vi "SaveBlock.vi"(6 "Registry":T13, 7 "start block":T21, 8 "error in (no error)":errorcluster, 9 "data":T9, 10 "data event config":T17, 11 "data event":T1) -> (0 "error out":errorcluster, 1 "file complete":bool, 2 "data event config out":T17, 3 "data event out":T1)   [LabVIEW 2017, in "CmsDataEventCreator.lvlib"]
uses:
  <vilib>/addons/InsightCM/Devices/Shared/Cms/CmsDataEventCreator/CmsDataEventCreator.lvlib
  <vilib>/addons/InsightCM/Devices/Shared/Common/DVRBuffer/controls/BufferLocation.ctl
  <vilib>/addons/InsightCM/Devices/Shared/Cms/CmsDataEventCreator/controls/DataEventConfig.ctl
  <vilib>/addons/InsightCM/Devices/Shared/Cms/CmsDataEventCreator/controls/AcqParams.ctl
  <vilib>/addons/InsightCM/Devices/Shared/Common/DataAccumulator/controls/AccumulationSettings.ctl
  <vilib>/addons/InsightCM/Devices/Shared/Common/DataAccumulator/controls/accumulationType.ctl
  <vilib>/addons/PointValueMap/controls/PointMap.ctl
  <vilib>/addons/InsightCM/Devices/Shared/Cms/CmsDataEventCreator/controls/GroupRegistry.ctl
  <vilib>/addons/InsightCM/Devices/Shared/Cms/CmsDataEventCreator/controls/DataSetRegistry.ctl
  <vilib>/addons/InsightCM/Devices/Shared/Common/DataEvent/controls/DataSetType.ctl
  <vilib>/addons/InsightCM/Devices/Shared/Common/DataEventCreator/controls/Registry_Trend.ctl
  <vilib>/addons/InsightCM/Devices/Shared/Common/DataFlow/controls/Data.ctl
  <vilib>/addons/InsightCM/Utilities/DataAccessors/controls/wfmSGL_DVR.ctl
  <vilib>/addons/InsightCM/Devices/Shared/Common/DataFlow/controls/Type.ctl
  <vilib>/addons/InsightCM/Devices/Shared/Common/DataEvent/controls/Event.ctl
  <vilib>/addons/InsightCM/MessageBus/Base/controls/DataEvent.ctl
  <vilib>/addons/InsightCM/MessageBus/Base/controls/KeyValuePair.ctl
  <vilib>/addons/InsightCM/Devices/Shared/Common/DataEvent/controls/DataSet.ctl
  <vilib>/addons/InsightCM/MessageBus/Base/controls/DataSetMetadata.ctl
  <vilib>/addons/InsightCM/MessageBus/Base/controls/TrendPoint.ctl
  <vilib>/addons/InsightCM/MessageBus/Base/controls/TrendAlarmUpdate.ctl
  <vilib>/addons/InsightCM/MessageBus/Base/controls/TrendAlarmTransition.ctl
  <vilib>/addons/InsightCM/Devices/Shared/Common/DataAccumulator/controls/DataStoreType.ctl
  <vilib>/addons/InsightCM/Utilities/Analysis/Shared/controls/PulsePositions.ctl
  <vilib>/addons/InsightCM/Devices/Shared/Common/DataAccumulator/DataAccumulator.lvlib
  <vilib>/addons/InsightCM/Utilities/Analysis/Shared/AnalysisHelper.lvlib
  <vilib>/addons/InsightCM/Devices/Shared/Common/DVRBuffer/DVRBuffer.lvlib
  <vilib>/addons/InsightCM/Devices/Shared/Common/DataFlow/DataFlow.lvlib
  <vilib>/addons/PointValueMap/PointValueMap.lvlib
  <vilib>/addons/InsightCM/Devices/Shared/Common/DataEvent/DataEvent.lvlib
  <vilib>/addons/InsightCM/Devices/Shared/Common/DataEventCreator/DataEventCreator.lvlib
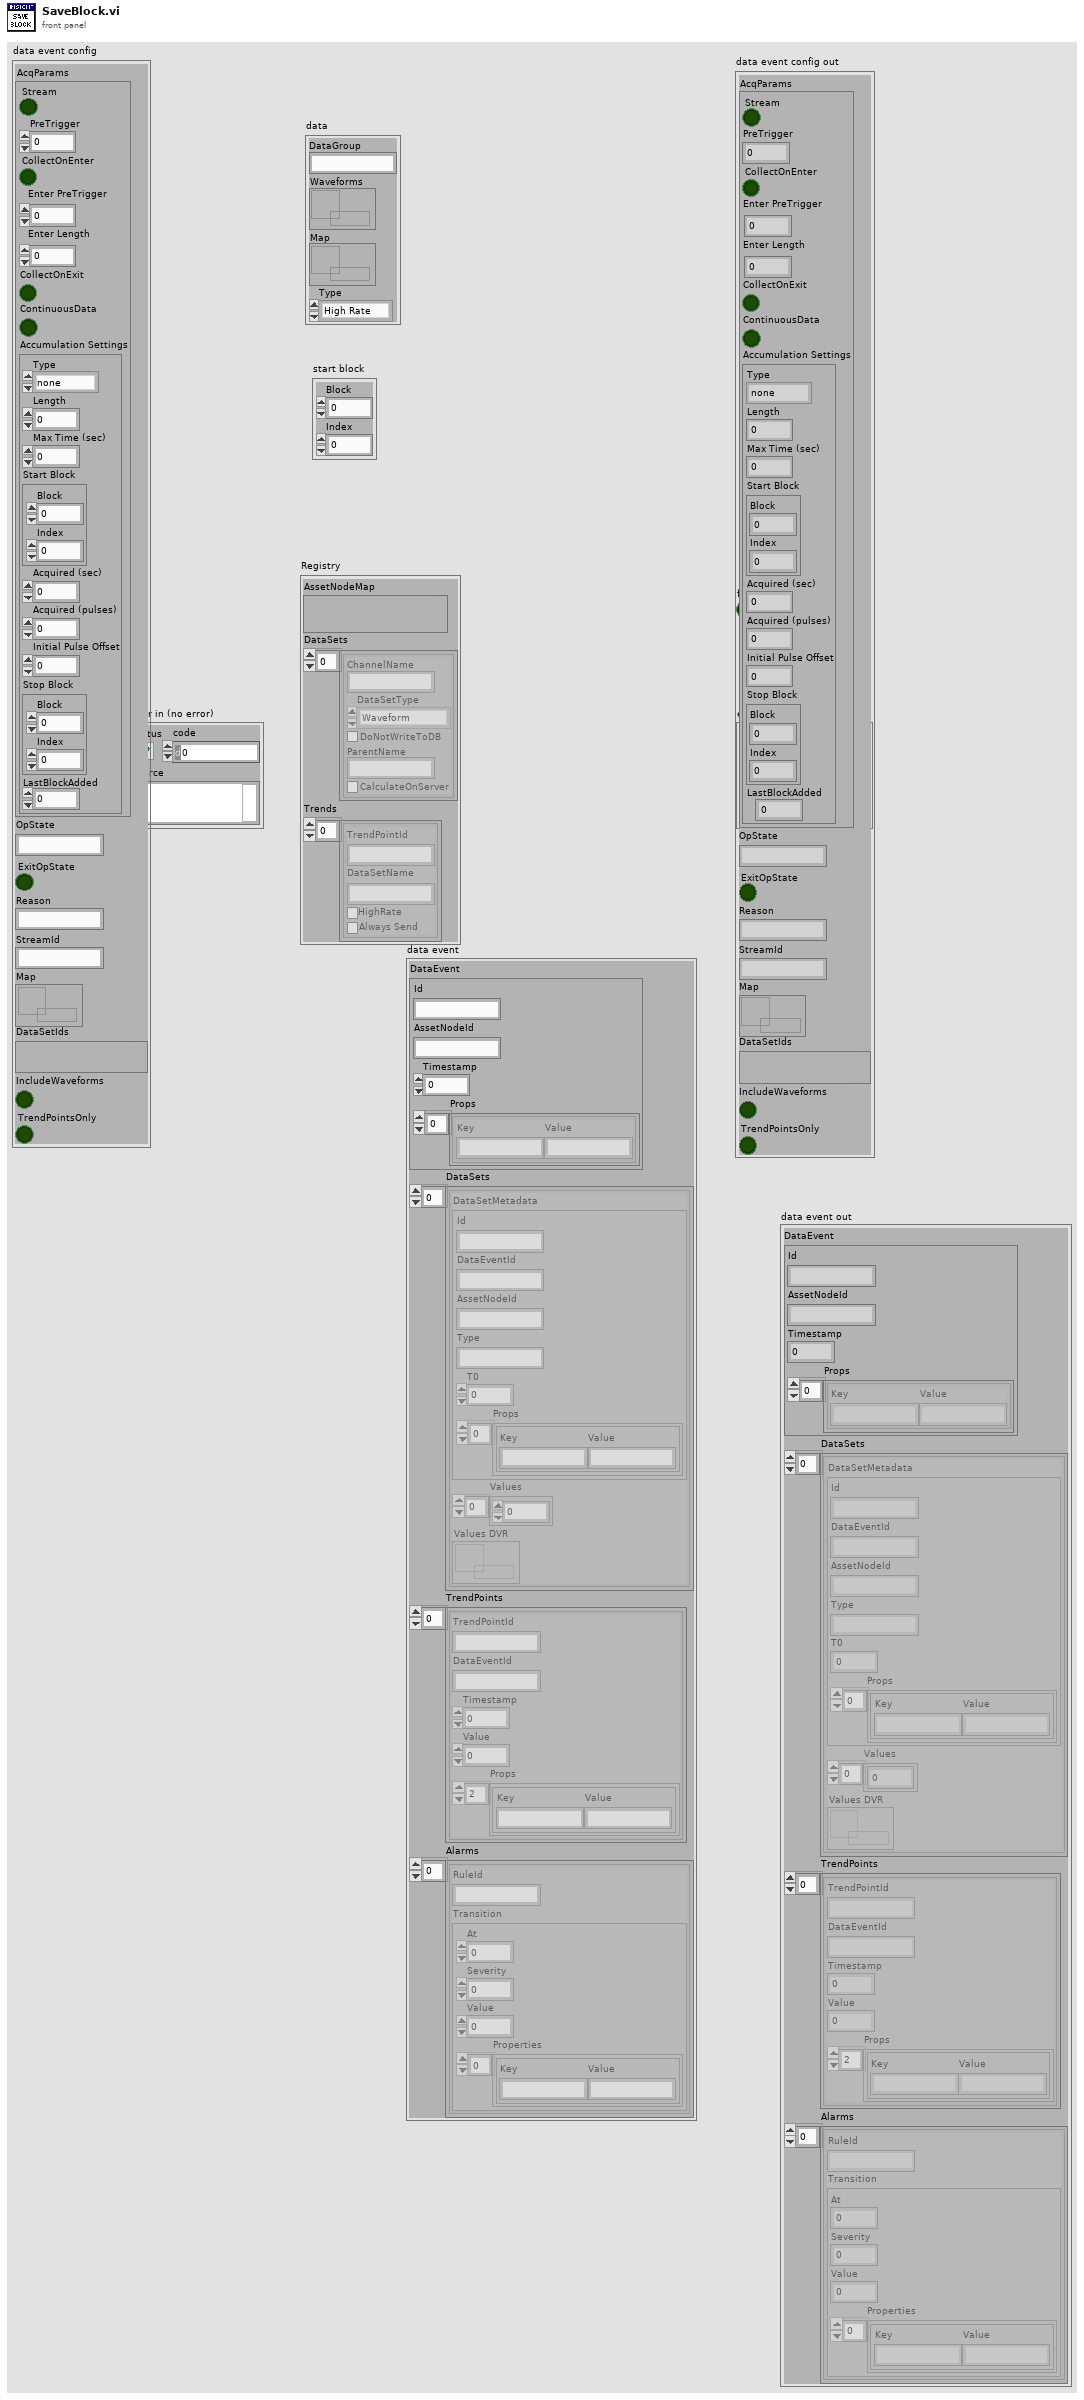
[diagram p1: front panel]
types:
  T1 = typedef "DataEvent.lvlib/Event.ctl" = cluster{"DataEvent":T2, "DataSets":T4[], "TrendPoints":T6[], "Alarms":T7[]}
  T2 = typedef "DataEvent.ctl" = cluster{"Id":string, "AssetNodeId":string, "Timestamp":i64, "Props":T3[]}
  T3 = typedef "KeyValuePair.ctl" = cluster{"Key":string, "Value":string}
  T4 = typedef "DataEvent.lvlib/DataSet.ctl" = cluster{"DataSetMetadata":T5, "Values":sgl[], "Values DVR":refnum<data-value>}
  T5 = typedef "DataSetMetadata.ctl" = cluster{"Id":string, "DataEventId":string, "AssetNodeId":string, "Type":string, "T0":i64, "Props":T3[]}
  T6 = typedef "TrendPoint.ctl" = cluster{"TrendPointId":string, "DataEventId":string, "Timestamp":i64, "Value":dbl, "Props":T3[]}
  T7 = typedef "TrendAlarmUpdate.ctl" = cluster{"RuleId":string, "Transition":T8}
  T8 = typedef "TrendAlarmTransition.ctl" = cluster{"At":i64, "Severity":i32, "Value":dbl, "Properties":T3[]}
  T9 = typedef "DataFlow.lvlib/Data.ctl" = cluster{"DataGroup":string, "Waveforms":T10, "Map":T11, "Type":T12}
  T10 = typedef "wfmSGL_DVR.ctl" = refnum<data-value>
  T11 = typedef "PointValueMap.lvlib/PointMap.ctl" = refnum<data-value>
  T12 = typedef "DataFlow.lvlib/Type.ctl" = enum16{"High Rate", "Low Rate", "Burst Mode"}
  T13 = typedef "CmsDataEventCreator.lvlib/GroupRegistry.ctl" = cluster{"AssetNodeMap":variant, "DataSets":T14[], "Trends":T16[]}
  T14 = typedef "CmsDataEventCreator.lvlib/DataSetRegistry.ctl" = cluster{"ChannelName":string, "DataSetType":T15, "DoNotWriteToDB":bool, "ParentName":string, "CalculateOnServer":bool}
  T15 = typedef "DataEvent.lvlib/DataSetType.ctl" = enum16{"Waveform", "SpeedProfile", "ThermalImage", "EmsaSweep"}
  T16 = typedef "DataEventCreator.lvlib/Registry_Trend.ctl" = cluster{"TrendPointId":string, "DataSetName":string, "HighRate":bool, "Always Send":bool}
  T17 = typedef "CmsDataEventCreator.lvlib/DataEventConfig.ctl" = cluster{"AcqParams":T18, "OpState":string, "ExitOpState":bool, "Reason":string, "StreamId":string, "Map":T11, "DataSetIds":variant, "IncludeWaveforms":bool, "TrendPointsOnly":bool}
  T18 = typedef "CmsDataEventCreator.lvlib/AcqParams.ctl" = cluster{"Stream":bool, "PreTrigger":i32, "CollectOnEnter":bool, "Enter PreTrigger":i32, "Enter Length":dbl, "CollectOnExit":bool, "ContinuousData":bool, "Accumulation Settings":T19}
  T19 = typedef "DataAccumulator.lvlib/AccumulationSettings.ctl" = cluster{"Type":T20, "Length":dbl, "Max Time (sec)":dbl, "Start Block":T21, "Acquired (sec)":dbl, "Acquired (pulses)":i32, "Initial Pulse Offset":dbl, "Stop Block":T21, "LastBlockAdded":u32}
  T20 = typedef "DataAccumulator.lvlib/accumulationType.ctl" = enum16{"none", "seconds", "revolutions"}
  T21 = typedef "DVRBuffer.lvlib/BufferLocation.ctl" = cluster{"Block":u32, "Index":i32}
  T22 = typedef "DataAccumulator.lvlib/DataStoreType.ctl" = cluster{"Group":string, "waveforms":waveform(sgl)[], "pulse positions array":T23[], "start block":T21}
  T23 = typedef "AnalysisHelper.lvlib/PulsePositions.ctl" = cluster{"Name":string, "Pulse Position Data":dbl[], "Pulses Per Rev":i32}
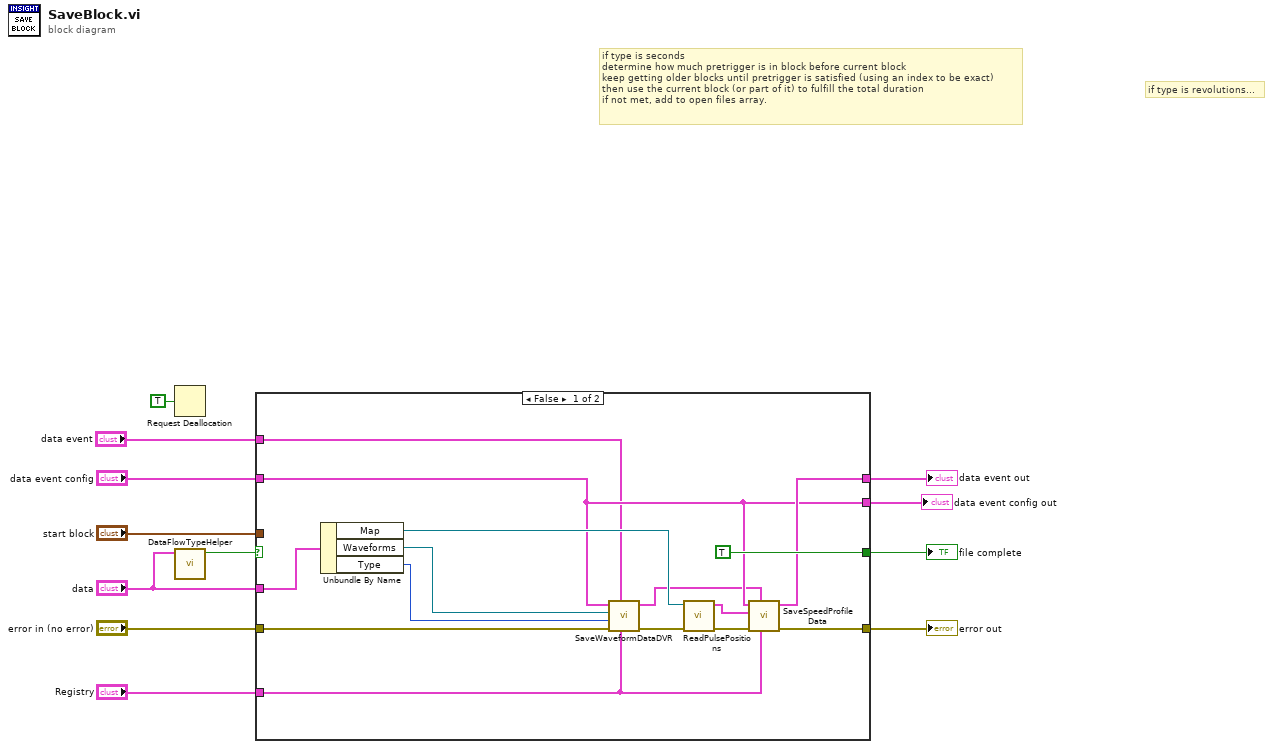
[diagram p0: block diagram]
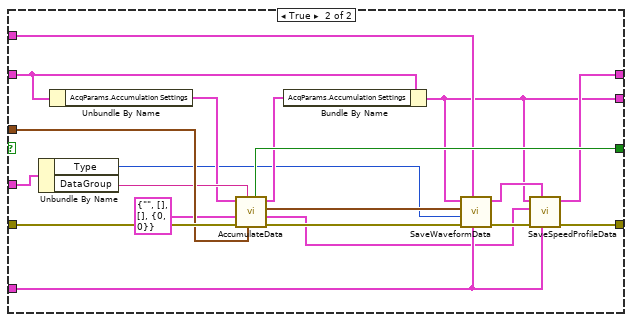
[diagram p2: hidden frame]
diagram:
  # "if type is revolutions..."
  # "if type is seconds\ndetermine how much pretrigger is in block before current block\nkeep getting older blocks until pretrigger is satisfied (using an index to be exact)\nthen use the current block (or part of it) to fulfill the total duration\nif not met, add to open files array."
  n1 = Request Deallocation(TRUE ("flag")) -> ()
  n2 = call <vilib>:"DataFlowTypeHelper.vi"("data"="data") -> ("high rate"=w2:bool)  [unwired: 8 in, 2 out]
  n3 = case shown="False" w2 {
    tunnel: "error in (no error)" -> [w18 w46]
    tunnel: "data event config" -> [w17 w33]
    tunnel: "Registry" -> [w16 w38]
    tunnel: [w23 w34] -> w4
    tunnel: "start block" -> [_ w45]
    tunnel: [TRUE ("file complete") w43] -> w8
    tunnel: [w22 w35] -> w7
    tunnel: "data" -> [w27 w47]
    tunnel: "data event" -> [w15 w31]
    tunnel: [w17 w29] -> w5
    frame False {
      n4 = Unbundle By Name(w27) -> ("Map"=w21:T11, "Waveforms"=w20:T10, "Type"=w19:T12)
      n5 = call <vilib>:"SaveWaveformDataDVR.vi"("Registry"=w16, "data event data"=w15, "error in (no error)"=w18, "dataflow type"=w19, "Waveforms"=w20, "data event"=w17) -> ("error out"=w13:errorcluster, "data event data out"=w14:T1)  [unwired: 4 in]
      n6 = call <vilib>:"ReadPulsePositions.vi"("error in (no error)"=w13, "Map"=w21) -> ("error out"=w25:errorcluster, "pulse positions array"=w26:T23[])  [unwired: 7 in, 1 out]
      n7 = call <vilib>:"SaveSpeedProfileData.vi"("registry"=w16, "data event data"=w14, "error in (no error)"=w25, "pulse positions array"=w26, "data event config"=w17) -> ("error out"=w22:errorcluster, "data event data out"=w23:T1)  [unwired: 5 in]
    }
    frame True {
      n8 = Unbundle By Name(w47) -> ("Type"=w28:T12, "DataGroup"=w44:string)
      n9 = Unbundle By Name(w33) -> ("AcqParams.Accumulation Settings"=w42:T19)
      n10 = call <vilib>:"AccumulateData.vi"("new block"=w45, "data group"=w44, "error in (no error)"=w46, "data in"=T22 {"Group"="", "waveforms"=[], "pulse positions array"=[], "start block"={"Block"=0, "Index"=0}}, "accumulation settings"=w42) -> ("error out"=w39:errorcluster, "pulse positions array"=w36:T23[], "waveforms"=w40:waveform(sgl)[], "accumulation settings out"=w41:T19, "accumulation complete"=w43:bool)  [unwired: 1 in, 1 out]
      n11 = Bundle By Name(cluster=w33, "AcqParams.Accumulation Settings"=w41) -> (w29:T17)
      n12 = call <vilib>:"SaveWaveformData.vi"("Registry"=w38, "data event data"=w31, "error in (no error)"=w39, "dataflow type"=w28, "waveforms"=w40, "data event"=w29) -> ("error out"=w37:errorcluster, "data event data out"=w30:T1)  [unwired: 4 in]
      n13 = call <vilib>:"SaveSpeedProfileData.vi"("registry"=w38, "data event data"=w30, "error in (no error)"=w37, "pulse positions array"=w36, "data event config"=w29) -> ("error out"=w35:errorcluster, "data event data out"=w34:T1)  [unwired: 5 in]
    }
  }
  "error out" <- w7
  "file complete" <- w8
  "data event config out" <- w5
  "data event out" <- w4
